vi "average_column_of_matrix.vi"() -> ()   [LabVIEW 2021]
uses:
  <vilib>/Analysis/Matrix/Datatypes/RealMatrix.ctl
  <vilib>/Analysis/Matrix/NI_Matrix.lvlib
panel:
  out "output":dbl[][](array[numeric])
  in  "loops":dbl
  in  "col index":dbl
  in  "blank":dbl[](array[numeric])
  in  "mat":T1
  out "avg":dbl
  out "num":dbl
  out "sum":dbl
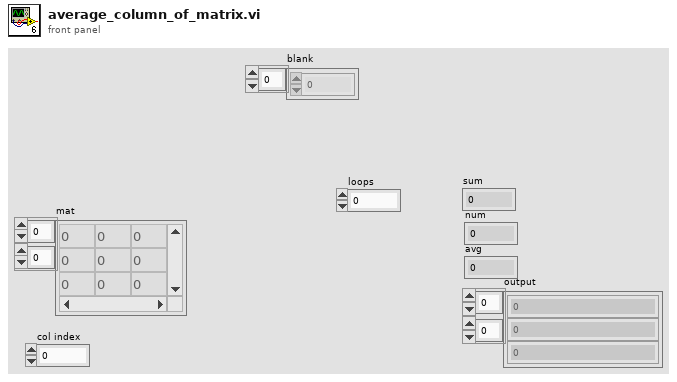
[diagram p1: front panel]
types:
  T1 = typedef "NI_Matrix.lvlib/RealMatrix.ctl" = dbl[][]
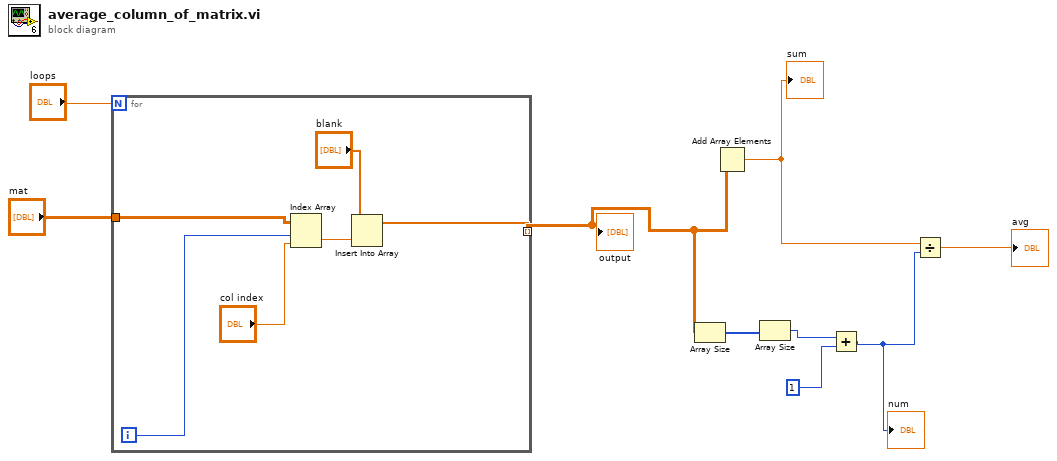
[diagram p0: block diagram]
diagram:
  n1 = for {
    N: "loops" -> [_]
    tunnel: [w11] -> w6 mode=indexing
    tunnel: "mat" -> [w10]
    i -> [w12]
    n2 = Index Array(array=w10, index (row)=w12, index (col)="col index") -> (element=w14:dbl)
    n3 = Insert Into Array(array="blank", new element=w14) -> (w11:dbl[])  [unwired: 1 in]
  }
  "output" <- w6
  n4 = Array Size(array=w6) -> (size(s)=w5:i32[])
  n5 = Add Array Elements(numeric array=w6) -> (sum=w9:dbl)
  "sum" <- w9
  n6 = Array Size(array=w5) -> (size(s)=w3:i32)
  n7 = Add(x=w3, y=1) -> (x+y=w2:i32)
  "num" <- w2
  n8 = Divide(x=w9, y=w2) -> (x/y=→"avg":dbl)
